vi "BigIntToHexString.vi"(1 "a":cluster{"Boolean":bool, "Array":u64[]}) -> (0 "Hex string":string)   [LabVIEW 2023]
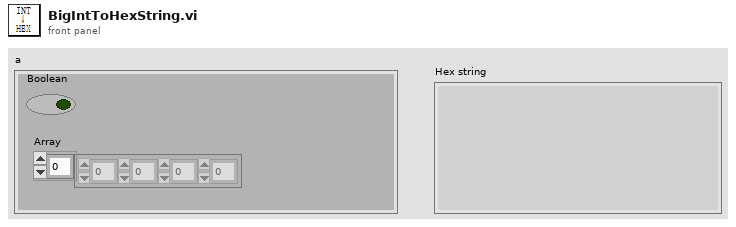
[diagram p1: front panel]
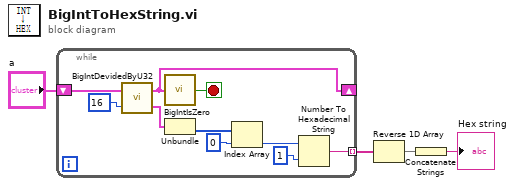
[diagram p0: block diagram]
diagram:
  n1 = while {
    shift-right: [w5] -> _
    shift-left: "a" -> [w14]
    tunnel: [w6] -> w3 mode=indexing
    stop <- w12 stop-if-true
    n2 = call "BigIntDevidedByU32.vi"("b (<1e9)"=u64 16, "a"=w14) -> ("a % b"=w11:cluster{"Boolean":bool, "Array":u64[]}, "a / b"=w5:cluster{"Boolean":bool, "Array":u64[]})
    n3 = call "BigIntIsZero.vi"("a"=w5) -> ("a = 0"=w12:bool)
    n4 = Unbundle(w11) -> ("Array"=w10:u64[])  [unwired: 1 out]
    n5 = Index Array(array=w10, index=0) -> (element=w8:u64)
    n6 = Number To Hexadecimal String(1:1, 2:w8) -> (0:w6:string)
  }
  n7 = Reverse 1D Array(array=w3) -> (reversed array=w1:string[])
  n8 = Concatenate Strings(w1) -> (→"Hex string":string)
